vi "Set Calibration (SubVI).vi"(11 "Calibration in":T1 {"Max Current A" format="%#_g mA"; "Max Current B" format="%#_g mA"; "UCL A" format="%#_g mA"; "LCL A" format="%#_g mA"; "UCL B" format="%#_g mA"; "LCL B" format="%#_g mA"}) -> (1 "Array":string[](array[string]))   [LabVIEW 2013]
uses:
  03 Type Def & Global/Calibration.ctl
  <vilib>/Utility/miscctls.llb/LVPointTypeDef.ctl
panel:
  in  "Cancel Button":bool
  in  "OK Button":bool
  in  "Calibration":T1 {"Max Current A" format="%#_g mA"; "Max Current B" format="%#_g mA"; "UCL A" format="%#_g mA"; "LCL A" format="%#_g mA"; "UCL B" format="%#_g mA"; "LCL B" format="%#_g mA"}
  # "Please change the calbration values as needed"
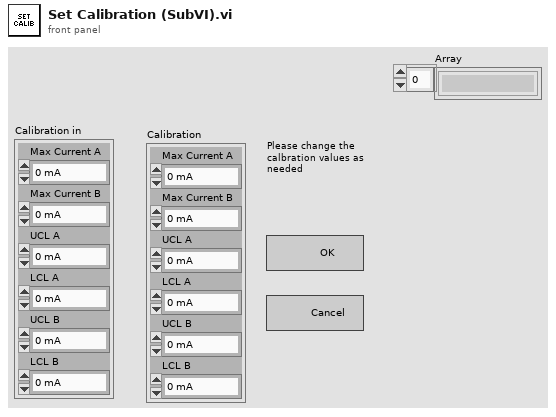
[diagram p1: front panel]
types:
  T1 = typedef "Calibration.ctl" = cluster{"Max Current A":dbl, "Max Current B":dbl, "UCL A":dbl, "UCL B":dbl, "LCL A":dbl, "LCL B":dbl}
  T2 = typedef "LVPointTypeDef.ctl" = cluster{"Horizontal":i16, "Vertical":i16}
  T3 = cluster{"Max Current A":bool, "Max Current B":bool, "UCL A":bool, "UCL B":bool, "LCL A":bool, "LCL B":bool}
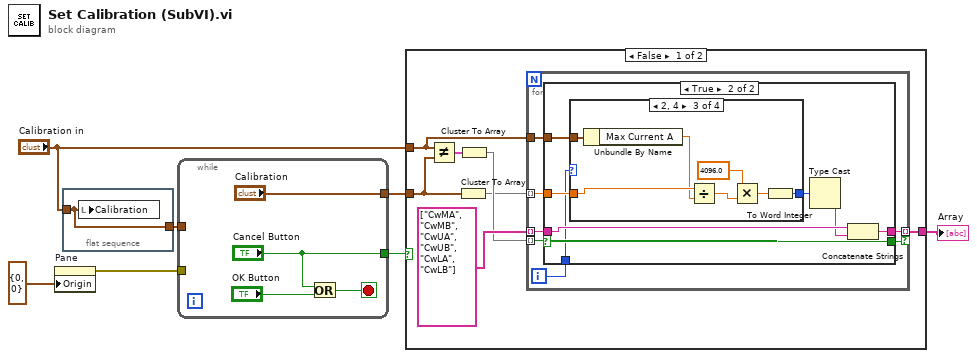
[diagram p0: block diagram]
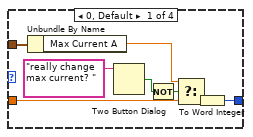
[diagram p3: hidden frame]
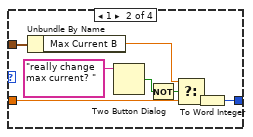
[diagram p4: hidden frame]
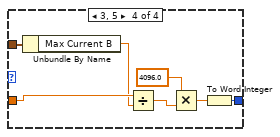
[diagram p5: hidden frame]
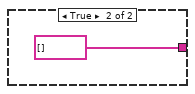
[diagram p6: hidden frame]
diagram:
  n1 = property on="Pane" class="Pane"("Origin"=T2 {"Horizontal"=0, "Vertical"=0}) -> (error out=w2:errorcluster)  [unwired: 2 in, 1 out]
  n2 = flat-sequence {
    tunnel: "Calibration in" -> [w8]
    tunnel: [w8] -> w1
    frame #0 {
      n3 = local write "Calibration"(w8) -> ()
    }
  }
  n4 = while {
    tunnel: ["Calibration"] -> w6
    tunnel: ["Cancel Button"] -> w5
    tunnel: w2 -> [_]
    tunnel: w1 -> [_]
    stop <- w12 stop-if-true
    n5 = Or(x="Cancel Button", y="OK Button") -> (x .or. y?=w12:bool)
  }
  n6 = case shown="False" w5 {
    tunnel: "Calibration in" -> [w13 _]
    tunnel: w6 -> [w15 _]
    tunnel: [w17 string[] []] -> w4
    frame False {
      n7 = Not Equal?(x=w13, y=w15) -> (x != y?=w16:T3)
      n8 = Cluster To Array(cluster=w15) -> (array=w14:dbl[])
      n9 = Cluster To Array(cluster=w16) -> (array=w18:bool[])
      n10 = for {
        tunnel: string[] ["CwMA", "CwMB", "CwUA", "CwUB", "CwLA", "CwLB"] -> [w24] mode=indexing
        tunnel: w18 -> [w26] mode=indexing
        tunnel: [w23] -> w17 mode=indexing if=w25
        tunnel: w14 -> [w22] mode=indexing
        tunnel: w13 -> [w20]
        i -> [w21]
        n11 = case shown="True" w26 {
          selector: w26 -> [w28 w36]
          tunnel: [w28 w36] -> w25
          tunnel: w24 -> [w27 w32]
          tunnel: [w27 w35] -> w23
          tunnel: w22 -> [_ w34]
          tunnel: w21 -> [_ w29]
          tunnel: w20 -> [_ w30]
          frame False {
          }
          frame True {
            n12 = case shown="2, 4" w29 {
              tunnel: w34 -> [w44 w52 w57 w64]
              tunnel: [w37 w45 w59 w66] -> w33
              tunnel: w30 -> [w42 w50 w58 w65]
              frame 0, Default {
                n13 = Unbundle By Name(w42) -> ("Max Current A"=w39:dbl)
                n14 = Two Button Dialog(message="really change max current? ") -> (T button?=w40:bool)  [unwired: 2 in]
                n15 = Not(x=w40) -> (.not. x?=w38:bool)
                n16 = Select(t=w39, s=w38, f=w44) -> (s? t:f=w41:dbl)
                n17 = To Word Integer(number=w41) -> (16bit integer=w37:i16)
              }
              frame 1 {
                n18 = Unbundle By Name(w50) -> ("Max Current B"=w47:dbl)
                n19 = Two Button Dialog(message="really change max current? ") -> (T button?=w48:bool)  [unwired: 2 in]
                n20 = Not(x=w48) -> (.not. x?=w46:bool)
                n21 = Select(t=w47, s=w46, f=w52) -> (s? t:f=w49:dbl)
                n22 = To Word Integer(number=w49) -> (16bit integer=w45:i16)
              }
              frame 2, 4 {
                n23 = Unbundle By Name(w58) -> ("Max Current A"=w56:dbl)
                n24 = Divide(x=w57, y=w56) -> (x/y=w54:dbl)
                n25 = Multiply(x=4096.0, y=w54) -> (x*y=w55:dbl)
                n26 = To Word Integer(number=w55) -> (16bit integer=w59:i16)
              }
              frame 3, 5 {
                n27 = Unbundle By Name(w65) -> ("Max Current B"=w63:dbl)
                n28 = Divide(x=w64, y=w63) -> (x/y=w61:dbl)
                n29 = Multiply(x=4096.0, y=w61) -> (x*y=w62:dbl)
                n30 = To Word Integer(number=w62) -> (16bit integer=w66:i16)
              }
            }
            n31 = Type Cast(x=w33) -> (*(type *) &x=w31:string)  [unwired: 1 in]
            n32 = Concatenate Strings(w32, w31) -> (w35:string)
          }
        }
      }
    }
    frame True {
    }
  }
  "Array" <- w4
